vi "SET HV SUPPLY MEASURE IV.vi"(0 "ORSAY":refnum<visa-resource-name>, 1 "SETTLE":i32, 2 "HV SUPPLY":u16(ring) items=["BEAM ENERGY", "EXTRACTOR", "SUPPRESSOR", "CONDENSOR", "OBJECTIVE"], 7 "VOLTAGE":dbl[unit], 11 "ORSAY ERROR":errorcluster, 12 "APPEND":string) -> (4 "ORSAY 2":refnum<visa-resource-name>, 15 "ORSAY ERROR":errorcluster)   [LabVIEW 2018]
panel:
  out "read buffer":string
  out "concatenated string":string
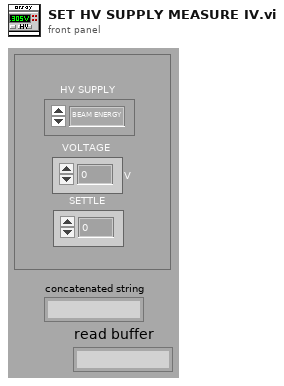
[diagram p1: front panel]
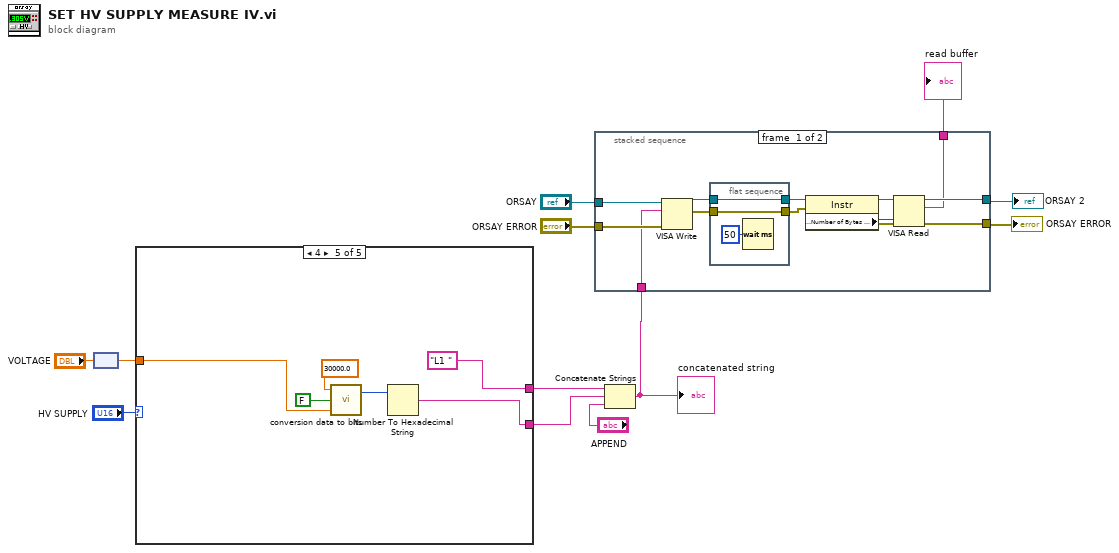
[diagram p0: block diagram]
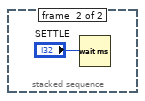
[diagram p2: hidden frame]
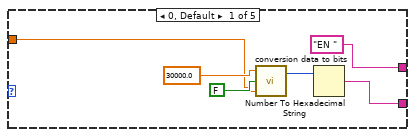
[diagram p3: hidden frame]
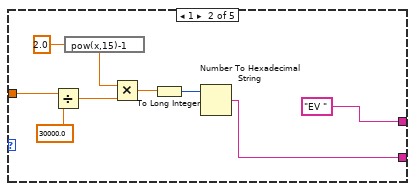
[diagram p4: hidden frame]
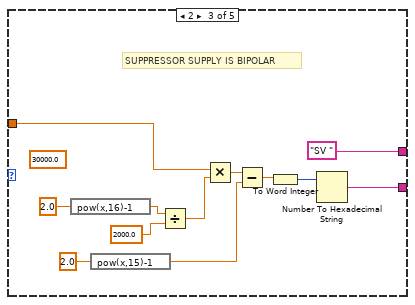
[diagram p5: hidden frame]
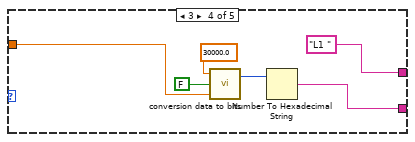
[diagram p6: hidden frame]
diagram:
  n1 = node("VOLTAGE") -> (w3:dbl)
  n2 = case shown="4" "HV SUPPLY" {
    tunnel: ["EN " "EV " "SV " "L1 " "L1 "] -> w8
    tunnel: w3 -> [w14 w25 w35 w43 w48]
    tunnel: [w13 w19 w28 w40 w46] -> w2
    frame 0, Default {
      n3 = call "conversion data to bits.vi"("Data input"=w14, "15 /16b"=FALSE, "Max supply"=sgl 30000.0) -> ("15 bits output"=w17:u16)  [unwired: 1 out]
      n4 = Number To Hexadecimal String(2:w17) -> (0:w13:string)  [unwired: 1 in]
    }
    frame 1 {
      n5 = Divide(x=w25, y=30000.0 ("Max supply")) -> (x/y=w24:dbl)
      n6 = expression code="pow(x,15)-1"(2.0) -> (w22:dbl)
      n7 = Multiply(x=w22, y=w24) -> (x*y=w21:dbl)
      n8 = To Long Integer(number=w21) -> (32bit integer=w20:i32)
      n9 = Number To Hexadecimal String(2:w20) -> (0:w19:string)  [unwired: 1 in]
    }
    frame 2 {
      (unwired) sgl 30000.0 ("Max supply")
      # "SUPPRESSOR SUPPLY IS BIPOLAR"
      n10 = expression code="pow(x,16)-1"(2.0) -> (w37:dbl)
      n11 = expression code="pow(x,15)-1"(2.0) -> (w31:dbl)
      n12 = Divide(x=w37, y=2000.0) -> (x/y=w34:dbl)
      n13 = Multiply(x=w35, y=w34) -> (x*y=w33:dbl)
      n14 = Subtract(x=w33, y=w31) -> (x-y=w30:dbl)
      n15 = To Word Integer(number=w30) -> (16bit integer=w29:i16)
      n16 = Number To Hexadecimal String(2:w29) -> (0:w28:string)  [unwired: 1 in]
    }
    frame 3 {
      n17 = call "conversion data to bits.vi"("Data input"=w43, "15 /16b"=FALSE, "Max supply"=sgl 30000.0) -> ("15 bits output"=w42:u16)  [unwired: 1 out]
      n18 = Number To Hexadecimal String(2:w42) -> (0:w40:string)  [unwired: 1 in]
    }
    frame 4 {
      n19 = call "conversion data to bits.vi"("Data input"=w48, "15 /16b"=FALSE, "Max supply"=sgl 30000.0) -> ("15 bits output"=w49:u16)  [unwired: 1 out]
      n20 = Number To Hexadecimal String(2:w49) -> (0:w46:string)  [unwired: 1 in]
    }
  }
  n21 = Concatenate Strings(w8, w2, "APPEND") -> (w9:string)
  "concatenated string" <- w9
  n22 = stacked-sequence {
    tunnel: "ORSAY" -> [w58 _]
    tunnel: "ORSAY ERROR" -> [w57 _]
    tunnel: w9 -> [w56 _]
    tunnel: [w53 _] -> w5
    tunnel: [w54 _] -> w6
    tunnel: [w52 _] -> w1
    frame #0 {
      n23 = VISA Write(VISA resource name=w58, write buffer=w56, error in (no error)=w57) -> (VISA resource name out=w55:refnum<visa-resource-name>, error out=w61:errorcluster)  [unwired: 1 out]
      n24 = flat-sequence {
        tunnel: [w67] -> w59
        tunnel: w55 -> [w67]
        tunnel: [w66] -> w60
        tunnel: w61 -> [w66]
        frame #0 {
          n25 = Wait (ms)(milliseconds to wait=u32 50) -> ()  [unwired: 1 out]
        }
      }
      n26 = property class="Instr"(reference=w59, error in=w60) -> (reference out=w64:refnum<visa-resource-name>, error out=w63:errorcluster, "Serial Settings:Number of Bytes at Serial Port"=w62:u32)
      n27 = VISA Read(VISA resource name=w64, byte count=w62, error in (no error)=w63) -> (VISA resource name out=w54:refnum<visa-resource-name>, read buffer=w52:string, error out=w53:errorcluster)  [unwired: 1 out]
    }
    frame #1 {
      n28 = Wait (ms)(milliseconds to wait="SETTLE") -> ()  [unwired: 1 out]
    }
  }
  "ORSAY 2" <- w6
  "ORSAY ERROR" <- w5
  "read buffer" <- w1
